vi "Picolog Open Device.vi"(6 "Mains Frequency":i16(ring) items=["50 Hz", "60 Hz"], 8 "Error In":errorcluster) -> (0 "Error Out":errorcluster, 3 "Instrument Handle Out":i16)   [LabVIEW 2017]
uses:
  usbtc08.dll
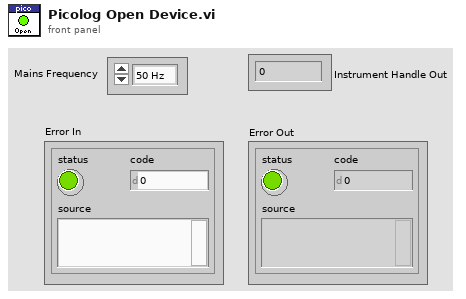
[diagram p1: front panel]
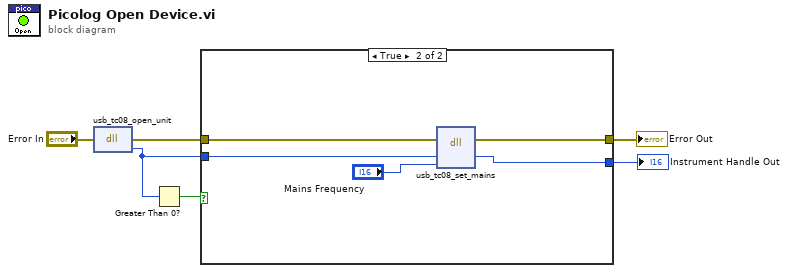
[diagram p0: block diagram]
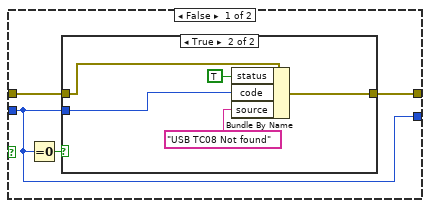
[diagram p2: hidden frame]
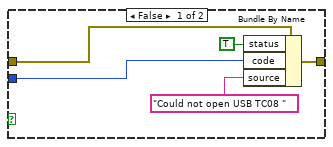
[diagram p3: hidden frame]
diagram:
  n1 = dll-call lib="usbtc08.dll" fn="usb_tc08_open_unit" label="OpenUnit"(error in="Error In") -> (error out=w6:errorcluster, "Handle"=w2:i16)  [unwired: 2 in, 1 out]
  n2 = Greater Than 0?(x=w2) -> (x > 0?=w1:bool)
  n3 = case shown="True" w1 {
    tunnel: w6 -> [w8 w25]
    tunnel: [w9 w24] -> w5
    tunnel: w2 -> [w7 w23]
    tunnel: [w7 w22] -> w4
    frame False {
      n4 = Equal To 0?(x=w7) -> (x = 0?=w10:bool)
      n5 = case shown="True" w10 {
        tunnel: [w14 w18] -> w9
        tunnel: w8 -> [w13 w20]
        tunnel: w7 -> [w12 w16]
        frame False {
          n6 = Bundle By Name(cluster=w13, "status"=TRUE, "code"=w12, "source"="Could not open USB TC08 ") -> (w14:errorcluster)
        }
        frame True {
          n7 = Bundle By Name(cluster=w20, "status"=TRUE, "code"=w16, "source"="USB TC08 Not found") -> (w18:errorcluster)
        }
      }
    }
    frame True {
      n8 = dll-call lib="usbtc08.dll" fn="usb_tc08_set_mains" label="Set Mains"(error in=w25, "Handle"=w23, "sixtyHertz"="Mains Frequency") -> (error out=w24:errorcluster, "Handle"=w22:i16)  [unwired: 4 in, 1 out]
    }
  }
  "Error Out" <- w5
  "Instrument Handle Out" <- w4
